vi "4.7.vi"() -> ()   [LabVIEW 2017]
panel:
  out "数值 2":dbl
  out "循环次数":i32
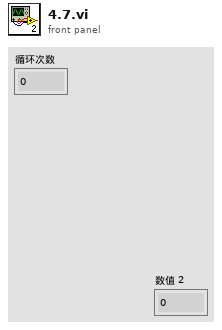
[diagram p1: front panel]
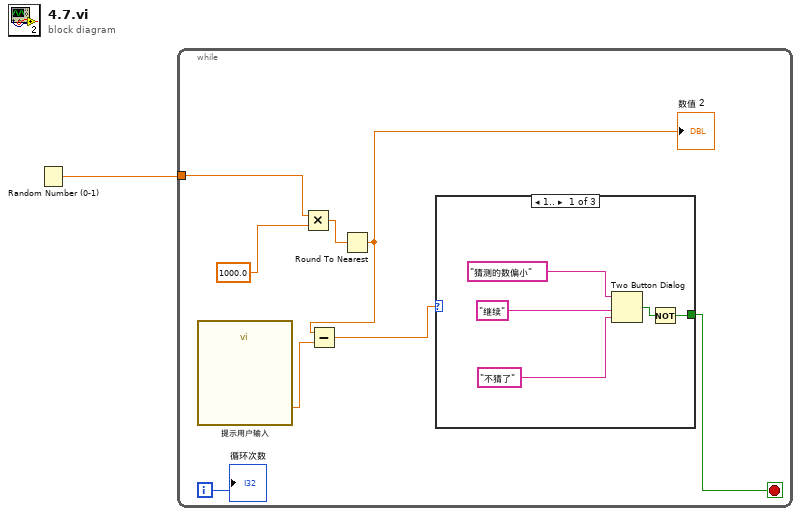
[diagram p0: block diagram]
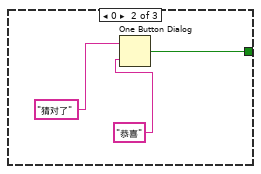
[diagram p2: hidden frame]
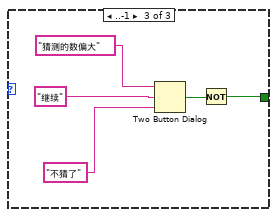
[diagram p3: hidden frame]
diagram:
  n1 = Random Number (0-1)() -> (number: 0 to 1=w1:dbl)
  n2 = while {
    tunnel: w1 -> [w2]
    i -> [w7]
    stop <- w3 stop-if-true
    n3 = call "提示用户输入"() -> ("请在1-1000内猜"=w5:dbl)  [unwired: 17 in, 2 out]
    n4 = Multiply(x=w2, y=1000.0 ("数字(0-1)")) -> (x*y=w8:dbl)
    n5 = Round To Nearest(number=w8) -> (nearest integer value=w6:dbl)
    "数值 2" <- w6
    n6 = Subtract(x=w6, y=w5) -> (x-y=w4:dbl)
    n7 = case shown="1.." w4 {
      tunnel: [w11 w16 w18] -> w3
      frame 1.. {
        n8 = Two Button Dialog(message="猜测的数偏小", 1:"不猜了", 2:"继续") -> (T button?=w10:bool)
        n9 = Not(x=w10) -> (.not. x?=w11:bool)
      }
      frame 0 {
        n10 = One Button Dialog(message="猜对了", button name ("OK")="恭喜") -> (true=w16:bool)
      }
      frame ..-1 {
        n11 = Two Button Dialog(message="猜测的数偏大", 1:"不猜了", 2:"继续") -> (T button?=w19:bool)
        n12 = Not(x=w19) -> (.not. x?=w18:bool)
      }
    }
    "循环次数" <- w7
  }
